vi "Controller Load Configuration From Parameters.vi"(8 "error in (no error)":errorcluster, 11 "FOFB Parameters":T1) -> (0 "error out":errorcluster, 3 "FOFB Configuration":T6)   [LabVIEW 2011, in "Controller VIs.lvlib"]
uses:
  Controller VIs.lvlib
  Types Definitions/Type FOFB Configuration.ctl
  Types Definitions/Type FOFB Parameters.ctl
  Types Definitions/Type Network Configuration.ctl
  Types Definitions/Type FA Configuration.ctl
  Types Definitions/Type Acquisition Network Configuration.ctl
  Types Definitions/Type Actuation Network Configuration.ctl
  XML VIs.lvlib
  Type Definitions.lvlib
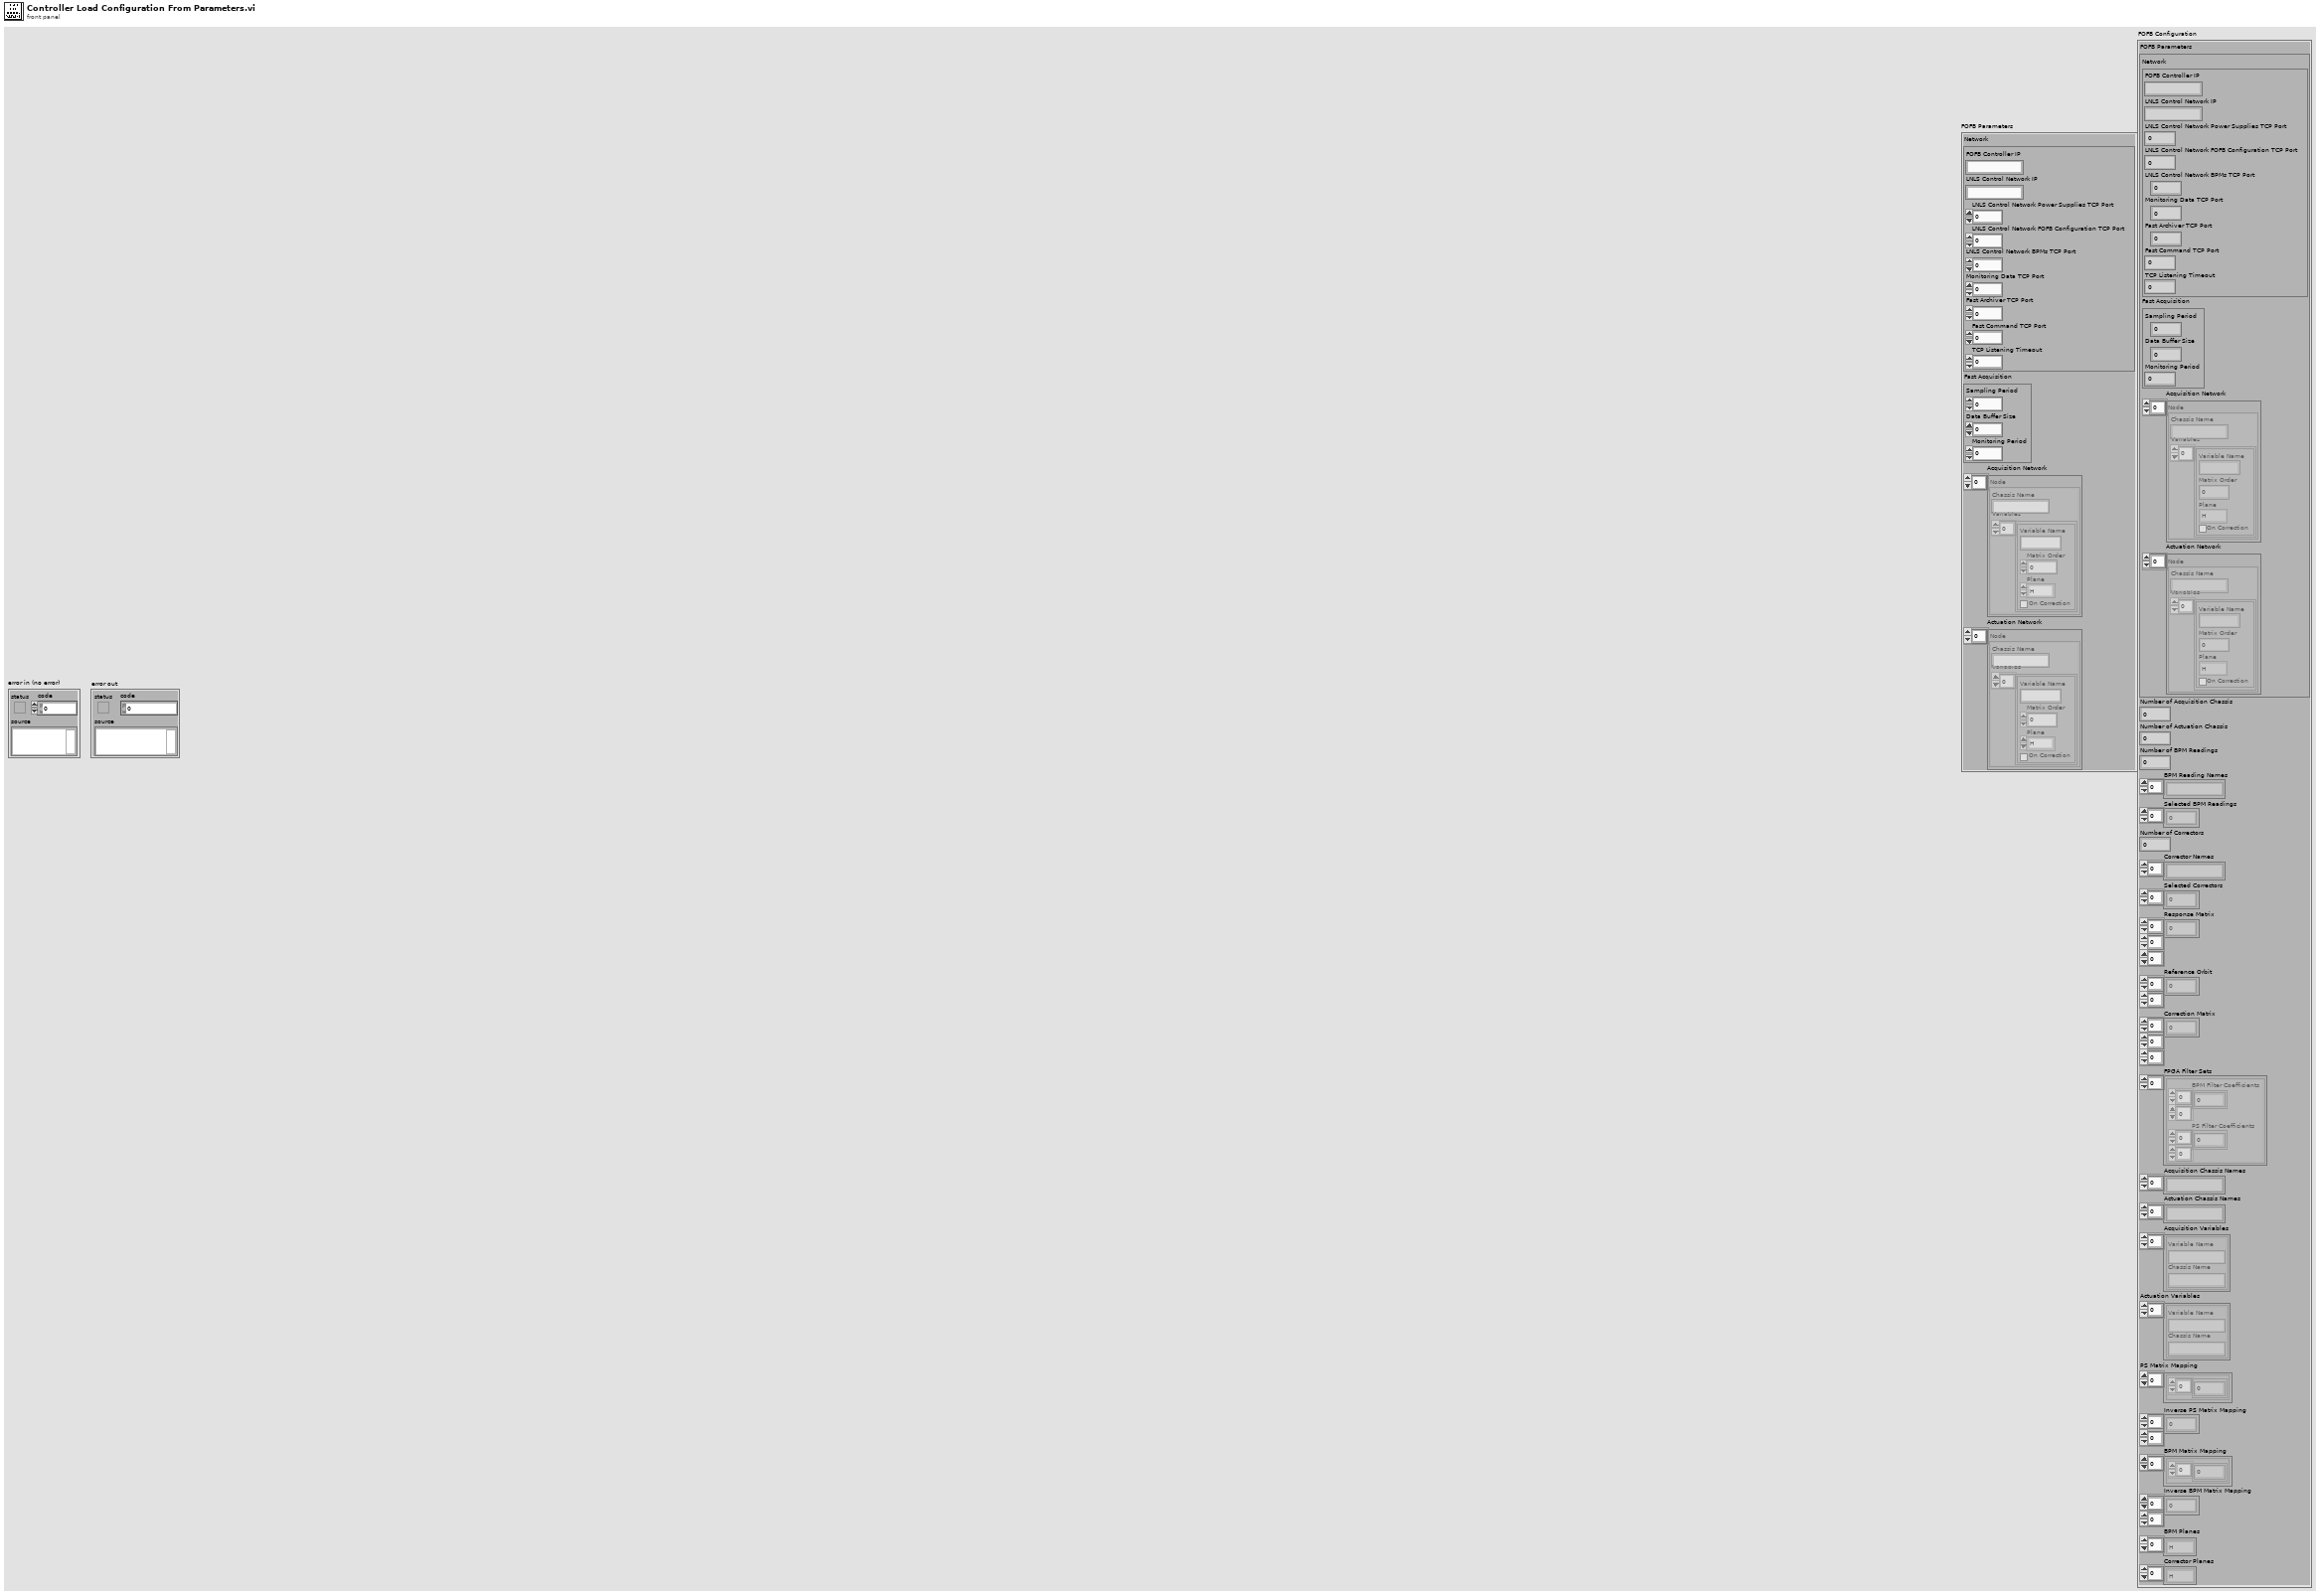
[diagram p1: front panel]
types:
  T1 = typedef "Type Definitions.lvlib/Type FOFB Parameters.ctl" = cluster{"Network":T2, "Fast Acquisition":T3, "Acquisition Network":T4, "Actuation Network":T5}
  T2 = typedef "Type Definitions.lvlib/Type Network Configuration.ctl" = cluster{"FOFB Controller IP":string, "LNLS Control Network IP":string, "LNLS Control Network Power Supplies TCP Port":u16, "LNLS Control Network FOFB Configuration TCP Port":u16, "LNLS Control Network BPMs TCP Port":u16, "Monitoring Data TCP Port":u16, "Fast Archiver TCP Port":u16, "Fast Command TCP Port":u16, "TCP Listening Timeout":i32}
  T3 = typedef "Type Definitions.lvlib/Type FA Configuration.ctl" = cluster{"Sampling Period":u32, "Data Buffer Size":u32, "Monitoring Period":u32}
  T4 = typedef "Type Definitions.lvlib/Type Acquisition Network Configuration.ctl" = cluster{"Chassis Name":string, "Variables":cluster{"Variable Name":string, "Matrix Order":u32, "Plane":enum8{"H", "V"}, "On Correction":bool}[]}[]
  T5 = typedef "Type Definitions.lvlib/Type Actuation Network Configuration.ctl" = cluster{"Chassis Name":string, "Variables":cluster{"Variable Name":string, "Matrix Order":u32, "Plane":enum8{"H", "V"}, "On Correction":bool}[]}[]
  T6 = typedef "Type Definitions.lvlib/Type FOFB Configuration.ctl" = cluster{"FOFB Parameters":T1, "Number of Acquisition Chassis":i32, "Number of Actuation Chassis":i32, "Number of BPM Readings":i32, "BPM Reading Names":string[], "Selected BPM Readings":u32[], "Number of Correctors":i32, "Corrector Names":string[], "Selected Correctors":u32[], "Response Matrix":dbl[][][], "Reference Orbit":dbl[][], "Correction Matrix":dbl[][][], "FPGA Filter Sets":cluster{"BPM Filter Coefficients":dbl[][], "PS Filter Coefficients":dbl[][]}[], "Acquisition Chassis Names":string[], "Actuation Chassis Names":string[], "Acquisition Variables":cluster{"Variable Name":string, "Chassis Name":string}[], "Actuation Variables":cluster{"Variable Name":string, "Chassis Name":string}[], "PS Matrix Mapping":cluster{u32[]}[], "Inverse PS Matrix Mapping":u32[][], "BPM Matrix Mapping":cluster{u32[]}[], "Inverse BPM Matrix Mapping":u32[][], "BPM Planes":enum8{"H", "V"}[], "Corrector Planes":enum8{"H", "V"}[]}
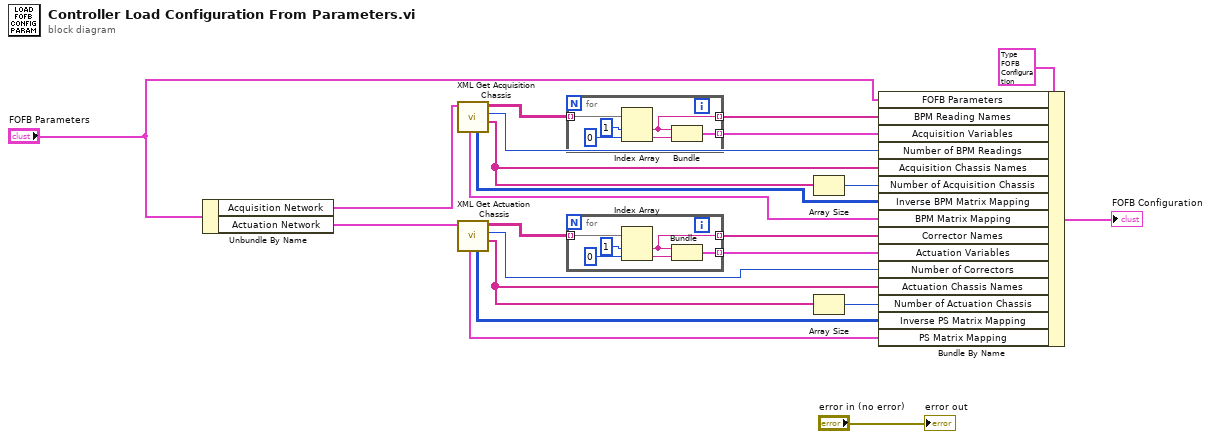
[diagram p0: block diagram]
diagram:
  n1 = Unbundle By Name("FOFB Parameters") -> ("Acquisition Network"=w2:T4, "Actuation Network"=w1:T5)
  n2 = call "XML Get Acquisition Chassis.vi"("Acquisition Network"=w2) -> ("Acquisition Chassis Names"=w11:string[], "Number of BPM Readings"=w17:i32, "Acquisition Variable Names"=w12:string[][], "Inverse BPM Matrix Mapping"=w20:u32[][], "BPM Matrix Mapping"=w21:cluster{u32[]}[])  [unwired: 4 in, 2 out]
  n3 = call "XML Get Actuation Chassis.vi"("Actuation Network"=w1) -> ("Actuation Chassis Names"=w7:string[], "Number of Correctors"=w15:i32, "Actuation Variable Names"=w5:string[][], "Inverse PS Matrix Mapping"=w8:u32[][], "PS Matrix Mapping"=w19:cluster{u32[]}[])  [unwired: 4 in, 2 out]
  n4 = for {
    tunnel: w12 -> [w27] mode=indexing
    tunnel: [w26] -> w14 mode=indexing
    tunnel: [w23] -> w13 mode=indexing
    n5 = Index Array(array=w27, index #1=1 ("index"), index #2=0 ("index")) -> (element #1=w23:string, element #2=w25:string)
    n6 = Bundle(w23, w25) -> (w26:cluster{string, string})  [unwired: 1 in]
  }
  n7 = for {
    tunnel: w5 -> [w33] mode=indexing
    tunnel: [w32] -> w6 mode=indexing
    tunnel: [w29] -> w10 mode=indexing
    n8 = Index Array(array=w33, index #1=1 ("index"), index #2=0 ("index")) -> (element #1=w29:string, element #2=w31:string)
    n9 = Bundle(w29, w31) -> (w32:cluster{string, string})  [unwired: 1 in]
  }
  n10 = Array Size(array=w11) -> (size(s)=w4:i32)
  n11 = Array Size(array=w7) -> (size(s)=w18:i32)
  n12 = Bundle By Name(cluster=T6 {"FOFB Parameters"={"Network"={"FOFB Controller IP"="", "LNLS Control Network IP"="", "LNLS Control Network Power Supplies TCP Port"=0, "LNLS Control Network FOFB Configuration TCP Port"=0, "LNLS Control Network BPMs TCP Port"=0, "Monitoring Data TCP Port"=0, "Fast Archiver TCP Port"=0, "Fast Command TCP Port"=0, "TCP Listening Timeout"=0}, "Fast Acquisition"={"Sampling Period"=0, "Data Buffer Size"=0, "Monitoring Period"=0}, "Acquisition Network"=[], "Actuation Network"=[]}, "Number of Acquisition Chassis"=0, "Number of Actuation Chassis"=0, "Number of BPM Readings"=0, "BPM Reading Names"=[], "Selected BPM Readings"=[], "Number of Correctors"=0, "Corrector Names"=[], "Selected Correctors"=[], "Response Matrix"=[], "Reference Orbit"=[], "Correction Matrix"=[], "FPGA Filter Sets"=[], "Acquisition Chassis Names"=[], "Actuation Chassis Names"=[], "Acquisition Variables"=[], "Actuation Variables"=[], "PS Matrix Mapping"=[], "Inverse PS Matrix Mapping"=[], "BPM Matrix Mapping"=[], "Inverse BPM Matrix Mapping"=[], "BPM Planes"=[], "Corrector Planes"=[]}, "FOFB Parameters"="FOFB Parameters", "BPM Reading Names"=w13, "Acquisition Variables"=w14, "Number of BPM Readings"=w17, "Acquisition Chassis Names"=w11, "Number of Acquisition Chassis"=w4, "Inverse BPM Matrix Mapping"=w20, "BPM Matrix Mapping"=w21, "Corrector Names"=w10, "Actuation Variables"=w6, "Number of Correctors"=w15, "Actuation Chassis Names"=w7, "Number of Actuation Chassis"=w18, "Inverse PS Matrix Mapping"=w8, "PS Matrix Mapping"=w19) -> (→"FOFB Configuration":T6)
  "error out" <- "error in (no error)"
